vi "Run.vi"(8 "error in (no error)":errorcluster caption="entrée d'erreur (pas d'erreur)", 11 "Swiss_Roll.lvclass":refnum<class "Swiss_Roll.lvclass">) -> (0 "error out":errorcluster caption="sortie d'erreur", 2 "Data":T1, 3 "Swiss_Roll.lvclass":refnum<class "Swiss_Roll.lvclass">)   [LabVIEW 2020, in "Swiss_Roll.lvclass"]
doc: "Returns :\n\nX : array of shape [n_samples, 3]\nThe points.\n\nt : array of shape [n_samples]\nThe univariate position of the sample according to the main dimension of the points in the manifold."
uses:
  Swiss_Roll.lvclass
  Swiss_Roll.lvclass/Swiss_Roll.ctl
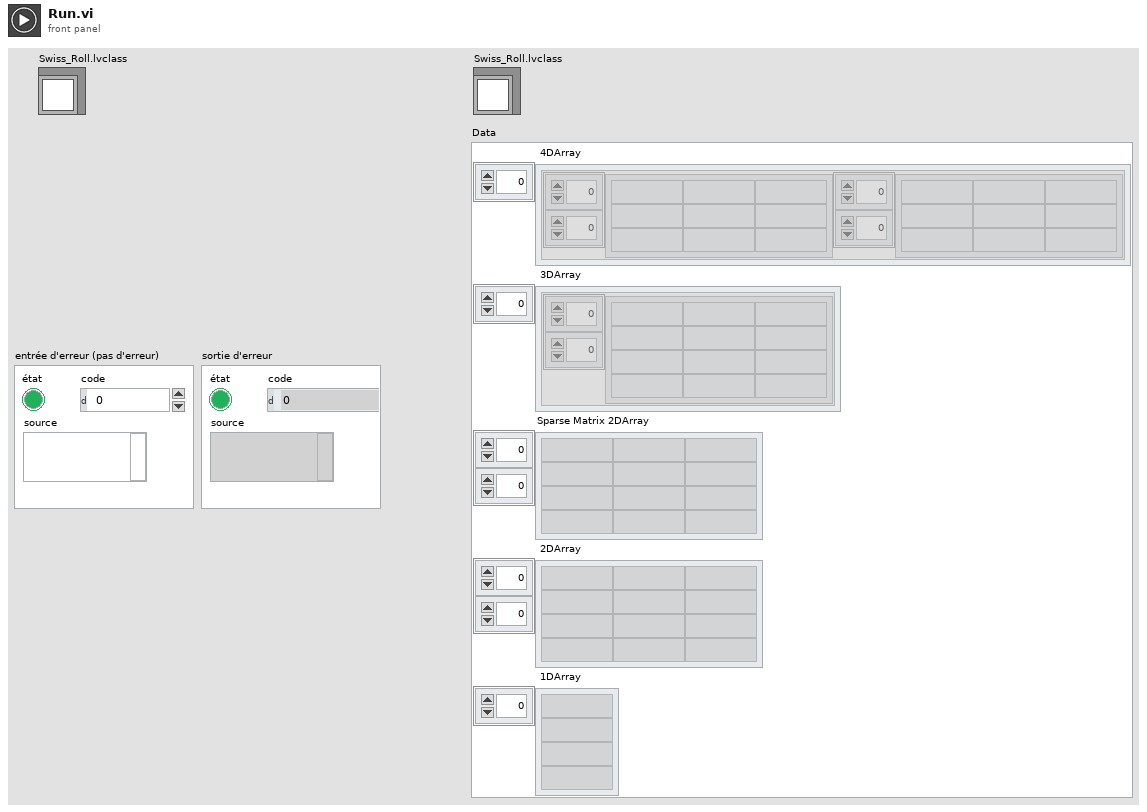
[diagram p1: front panel]
types:
  T1 = cluster{" 4DArray":cluster{"1":string[][], "2":string[][]}[], " 3DArray":cluster{"Tableau":string[][]}[], "Sparse Matrix 2DArray":string[][], " 2DArray":string[][], " 1DArray":string[]}
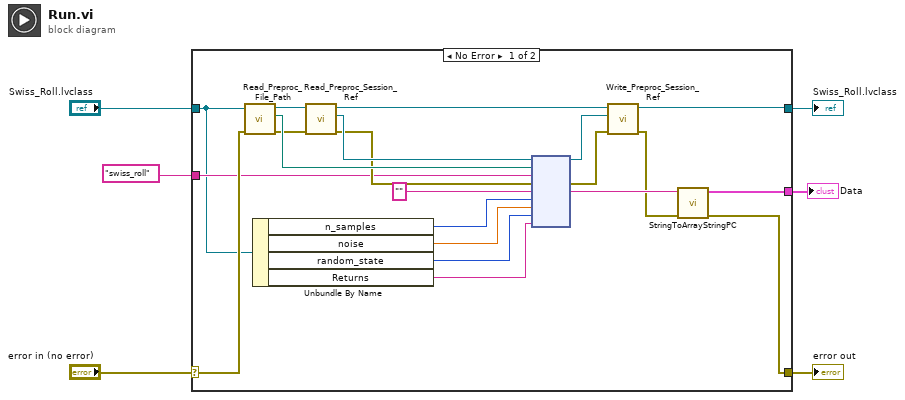
[diagram p0: block diagram]
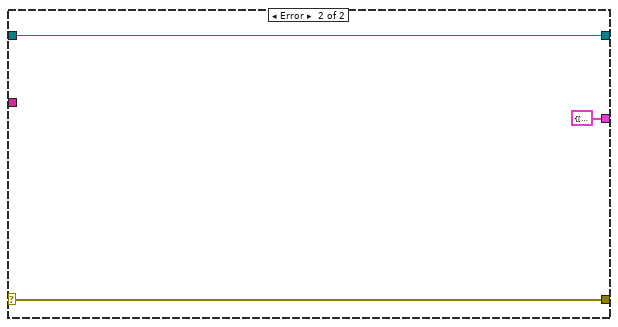
[diagram p2: hidden frame]
diagram:
  n1 = case shown="No Error" "error in (no error)" {
    selector: "error in (no error)" -> [w18 w30]
    tunnel: [w8 w30] -> w5
    tunnel: [w11 w29] -> w3
    tunnel: "Swiss_Roll.lvclass" -> [w16 w29]
    tunnel: "swiss_roll" -> [w17 _]
    tunnel: [w7 T1 {" 4DArray"=[], " 3DArray"=[], "Sparse Matrix 2DArray"=[], " 2DArray"=[], " 1DArray"=[]} ("Data")] -> w1
    frame No Error {
      n2 = call-dynamic "Read_Preproc_File_Path.vi"("error in (no error)"=w18, "Python in"=w16) -> ("error out"=w22:errorcluster, "File_Path"=w25:path, "Python out"=w27:refnum<class "Swiss_Roll.lvclass">)  [unwired: 7 in]
      n3 = Unbundle By Name(w16) -> ("n_samples"=w15:u32, "noise"=w14:dbl, "random_state"=w13:i32, "Returns"=w12:string)
      n4 = call-dynamic "Read_Preproc_Session_Ref.vi"("error in (no error)"=w22, "Python in"=w27) -> ("error out"=w23:errorcluster, "Session_ref"=w24:refnum<k35>, "Python out"=w26:refnum<class "Swiss_Roll.lvclass">)  [unwired: 7 in]
      n5 = node(w24, w25, w17, w23, "", w15, w14, w13, w12) -> (w19:refnum<k35>, w21:errorcluster, w10:string)  [unwired: 4 in, 2 out]
      n6 = call-dynamic "Write_Preproc_Session_Ref.vi"("error in (no error)"=w21, "Session_ref"=w19, "Python in"=w26) -> ("error out"=w9:errorcluster, "Python out"=w11:refnum<class "Swiss_Roll.lvclass">)  [unwired: 7 in]
      n7 = call "StringToArrayStringPC.vi"("sortie d'erreur"=w9, "Return value"=w10) -> ("sortie d'erreur"=w8:errorcluster, "Data"=w7:T1)  [unwired: 8 in]
    }
    frame Error {
    }
  }
  "error out" <- w5
  "Swiss_Roll.lvclass" <- w3
  "Data" <- w1
